vi "SetGrabberPosition.vi"(8 "error in":errorcluster, 10 "GrabberPosition":dbl, 11 "Robot_Interface in":refnum<class "Robot_Interface.lvclass">) -> (0 "error out":errorcluster, 3 "Robot_Interface out":refnum<class "Robot_Interface.lvclass">)   [LabVIEW 2015, in "Robot_Interface.lvclass"]
uses:
  Robot_Interface.lvclass
  Robot_Interface.lvclass/Robot_Interface.ctl
  Subsytems/JKI.Robot.SMO.Base/JKI.Robot.SMO.Base.lvclass
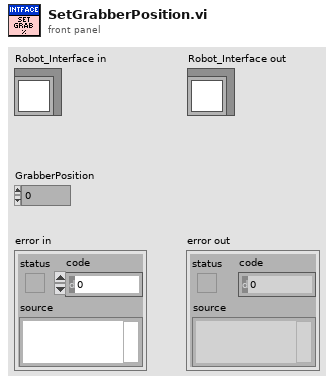
[diagram p1: front panel]
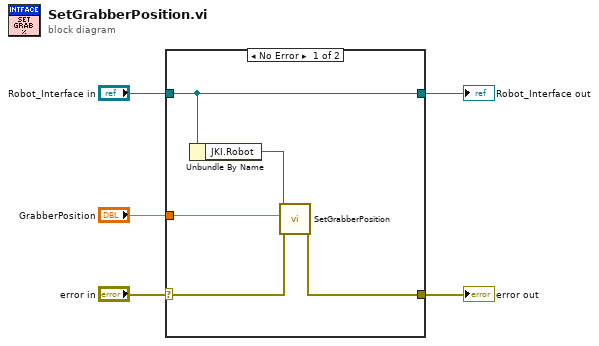
[diagram p0: block diagram]
diagram:
  n1 = case shown="No Error" "error in" {
    selector: "error in" -> [w8 w12]
    tunnel: [w7 w12] -> w4
    tunnel: [w6 w11] -> w2
    tunnel: "Robot_Interface in" -> [w6 w11]
    tunnel: "GrabberPosition" -> [w9 _]
    frame No Error {
      n2 = Unbundle By Name(w6) -> ("JKI.Robot"=w10:refnum<class "JKI.Robot.SMO.Base.lvclass">)
      n3 = call-dynamic "SetGrabberPosition.vi"("error in (no error)"=w8, "GrabberPosition"=w9, "JKI.Robot"=w10) -> ("error out"=w7:errorcluster)  [unwired: 7 in, 1 out]
    }
    frame Error {
    }
  }
  "error out" <- w4
  "Robot_Interface out" <- w2
